vi "GL_ProgramDownload.vi"(3 "error in":errorcluster, 4 "program":string, 5 "Galil.IGalil":refnum<k7>) -> (0 "error out":errorcluster, 1 "Uploaded Final":string, 2 "reference out":refnum<k7>)   [LabVIEW 2022 SP3]
panel:
  out "Initial Memory":string
  # "he vi downloads a porgram to the controller with the programDownload function.  It then uploads the program from the controller with the programUpload function and shows it on the front Panel"
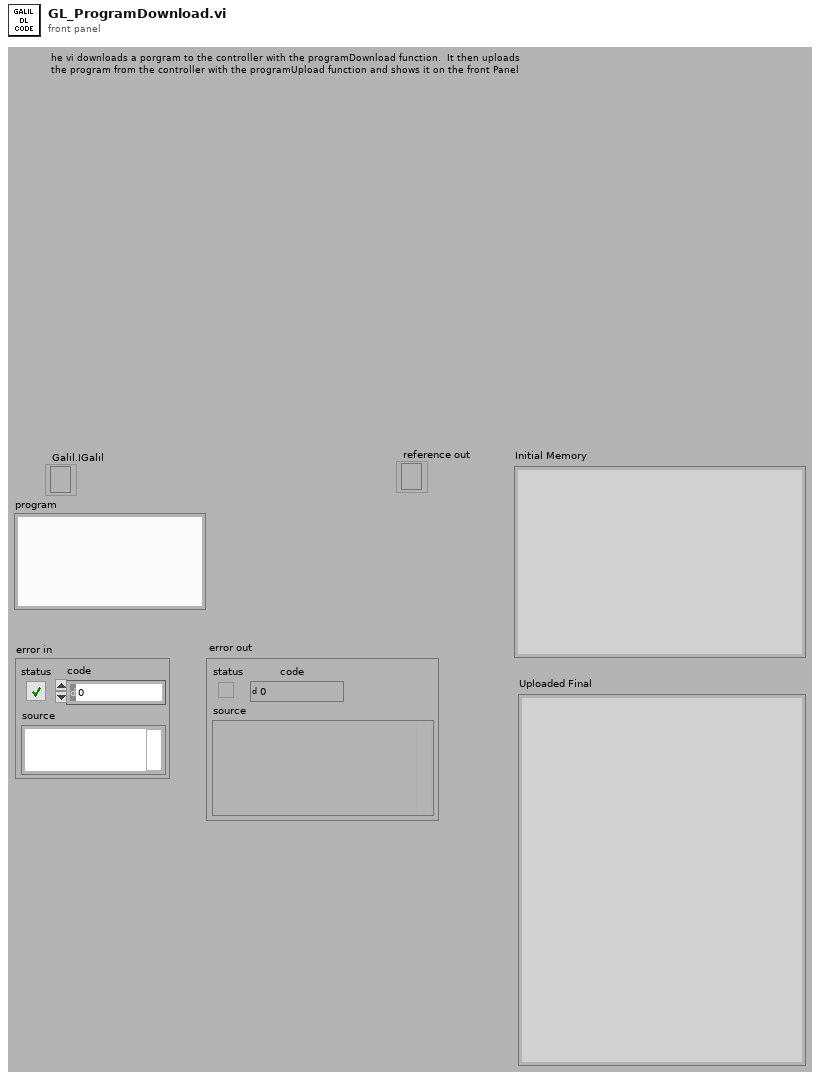
[diagram p1: front panel]
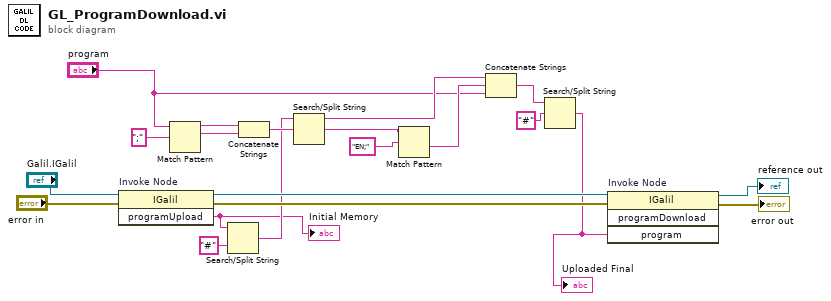
[diagram p0: block diagram]
diagram:
  n1 = invoke on="Invoke Node" class="IGalil" method="programUpload"(reference="Galil.IGalil", error in="error in") -> (reference out=w21:refnum<k7>, error out=w20:errorcluster, "programUpload"=w4:string)  [unwired: 1 in]
  "Initial Memory" <- w4
  n2 = Match Pattern(string="program", regular expression=";" ("search string/char (-)")) -> (before substring=w10:string, match substring=w9:string)  [unwired: 1 in, 2 out]
  n3 = Search/Split String(string=w4, search string/char (-)="#") -> (match + rest of string=w5:string)  [unwired: 1 in, 2 out]
  n4 = Concatenate Strings(w10, w9) -> (w8:string)
  n5 = Search/Split String(string=w5, search string/char (-)=w8) -> (substring before match=w15:string, match + rest of string=w14:string)  [unwired: 1 in, 1 out]
  n6 = Match Pattern(string=w14, regular expression="EN;") -> (after substring=w12:string)  [unwired: 1 in, 3 out]
  n7 = Concatenate Strings(w15, w12, "program") -> (w3:string)
  n8 = Search/Split String(string=w3, search string/char (-)="#") -> (match + rest of string=w2:string)  [unwired: 1 in, 2 out]
  "Uploaded Final" <- w2
  n9 = invoke on="Invoke Node" class="IGalil" method="programDownload"(reference=w21, error in=w20, "program"=w2) -> (reference out=→"reference out":refnum<k7>, error out=→"error out":errorcluster)  [unwired: 1 in, 2 out]
